vi "CLI.vi"() -> (0 "Error Out":errorcluster)   [LabVIEW 2019]
uses:
  BuildData.ctl
  <vilib>/AppBuilder/AB_API/common/AB_API Version Number.ctl
  <vilib>/regexp/Match Regular Expression.xnode
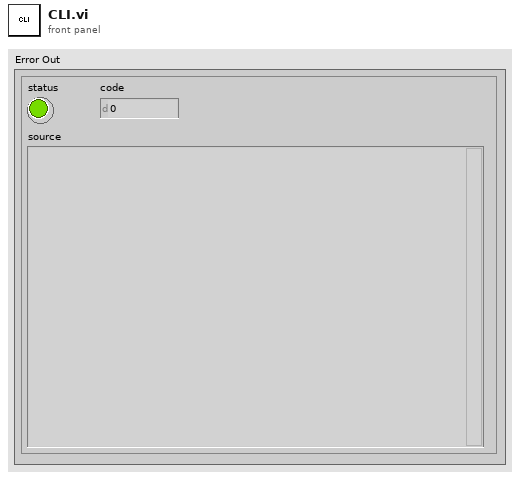
[diagram p1: front panel]
types:
  T1 = typedef "BuildData.ctl" = cluster{"Version number":T2, "Build Specification":string, "Project Path":path}
  T2 = typedef "AB_API Version Number.ctl" = cluster{"Major":u16, "Minor":u16, "Fix":u16, "Build":u16}
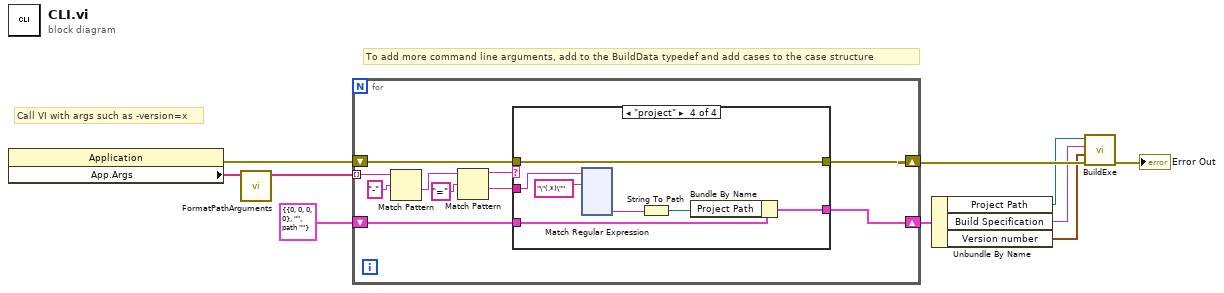
[diagram p0: block diagram]
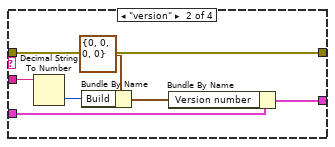
[diagram p3: hidden frame]
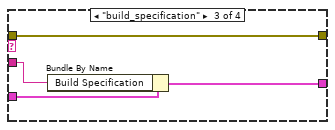
[diagram p4: hidden frame]
diagram:
  # "Call VI with args such as -version=x"
  # "To add more command line arguments, add to the BuildData typedef and add cases to the case structure"
  n1 = property class="Application"() -> (error out=w10:errorcluster, "App.Args"=w1:string[])  [unwired: 2 in, 1 out]
  n2 = call "FormatPathArguments.vi"("Arguments"=w1) -> ("Formatted Args"=w2:string[])  [unwired: 10 in]
  n3 = for {
    tunnel: w2 -> [w20] mode=indexing
    shift-right: [w13] -> w9
    shift-left: w10 -> [w14]
    shift-right: [w11] -> w6
    shift-left: T1 {"Version number"={"Major"=0, "Minor"=0, "Fix"=0, "Build"=0}, "Build Specification"="", "Project Path"=path ""} -> [w12]
    n4 = Match Pattern(string=w20, regular expression="-") -> (after substring=w18:string)  [unwired: 1 in, 3 out]
    n5 = Match Pattern(string=w18, regular expression="=") -> (before substring=w16:string, after substring=w15:string)  [unwired: 1 in, 2 out]
    n6 = case shown="\"project\"" w16 {
      tunnel: w15 -> [_ w29 w31 w36]
      tunnel: w14 -> [w22 w28 w30 w37]
      tunnel: [w22 w28 w30 w37] -> w13
      tunnel: w12 -> [w21 w24 w33 w39]
      tunnel: [w21 w23 w32 w38] -> w11
      frame Default {
        # "This case should never occur (I think...)"
      }
      frame "version" {
        n7 = Decimal String To Number(string=w29) -> (number=w27:i32)  [unwired: 2 in, 1 out]
        n8 = Bundle By Name(cluster=T2 {"Major"=0, "Minor"=0, "Fix"=0, "Build"=0} ("Version number"), "Build"=w27) -> (w25:T2)
        n9 = Bundle By Name(cluster=w24, "Version number"=w25) -> (w23:T1)
      }
      frame "build_specification" {
        n10 = Bundle By Name(cluster=w33, "Build Specification"=w31) -> (w32:T1)
      }
      frame "project" {
        n11 = xnode "Match Regular Expression"("input string"=w36, "regular expression"="\"(.*)\"") -> ("submatch 1"=w34:string)  [unwired: 4 in, 5 out]
        n12 = String To Path(string=w34) -> (path=w40:path)
        n13 = Bundle By Name(cluster=w39, "Project Path"=w40) -> (w38:T1)
      }
    }
  }
  n14 = Unbundle By Name(w6) -> ("Project Path"=w4:path, "Build Specification"=w5:string, "Version number"=w3:T2)
  n15 = call "BuildExe.vi"("Error In"=w9, "Version number"=w3, "Build specification name"=w5, "Path"=w4) -> ("Error Out"=→"Error Out":errorcluster)  [unwired: 7 in]
